vi "Get Property Data (U32).vi"(8 "error in":errorcluster, 10 "Property Name":string, 11 "Item Ref in":refnum<data-value>) -> (0 "error out":errorcluster, 3 "Property Value":u32)   [LabVIEW 2024, in "Config File Parser.lvlib" / "Property.lvclass"]
uses:
  Property.lvclass
  Property.lvclass/Property.ctl
  Item/Item.lvclass
  Property Type.ctl
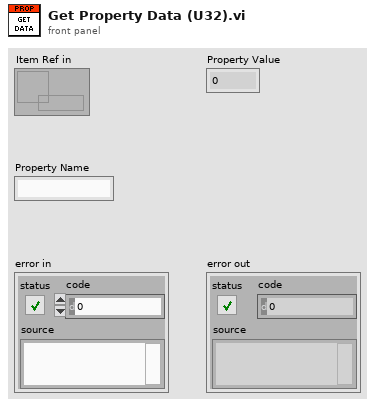
[diagram p1: front panel]
types:
  T1 = typedef "Config File Parser.lvlib/Property.lvclass/Property Type.ctl" = enum16{"Boolean", "Double", "String", "Path", "Dictionary", "DependentFile", "I16", "I32", "I64", "U16", "U32", "U64", "BooleanArray", "DoubleArray", "StringArray", "I16Array", "I32Array", "I64Array", "U16Array", "U32Array", "U64Array"}
  T2 = typedef "Config File Parser.lvlib/Item.lvclass/Item Type.ctl" = enum16{"Property", "Channel", "Section"}
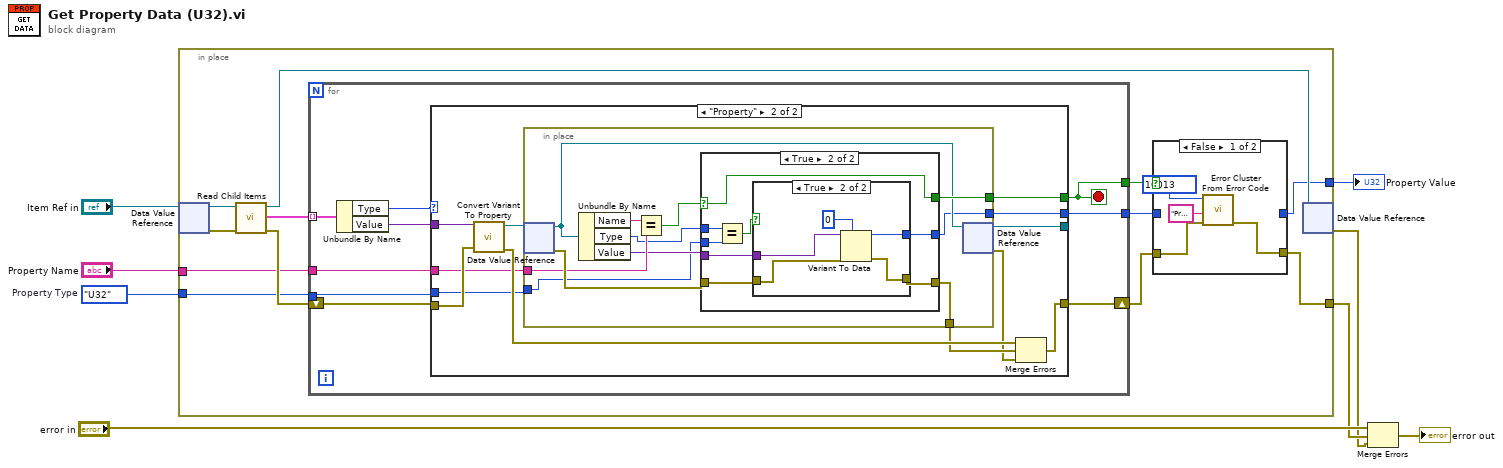
[diagram p0: block diagram]
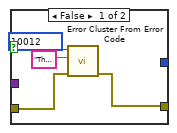
[diagram p5: hidden frame]
diagram:
  w2 = Property_Type."U32"  # Property Type
  n1 = in-place {
    in-place-border: "Property Name" -> [w14]
    in-place-border: w2 -> [w13]
    in-place-border: [w17] -> w7
    in-place-border: [w9] -> w1
    n2 = in-place-dvr #1("Item Ref in") -> (w16:refnum<class "Item.lvclass">, w20:errorcluster)
    n3 = call-dynamic "Read Child Items.vi"("error in"=w20, "Item in"=w16) -> ("error out"=w19:errorcluster, "Child Items"=w15:cluster{"Type":T2, "Value":variant}[], "Item out"=w12:refnum<class "Item.lvclass">)  [unwired: 7 in]
    n4 = for {
      tunnel: w15 -> [w33] mode=indexing
      tunnel: w14 -> [w30]
      tunnel: w13 -> [w29]
      shift-right: [w34] -> w18
      shift-left: w19 -> [w35]
      tunnel: [w28] -> w11
      tunnel: [w27] -> w10
      stop <- w28 stop-if-true
      n5 = Unbundle By Name(w33) -> ("Type"=w32:T2, "Value"=w31:variant)
      n6 = case shown="\"Property\"" w32 {
        tunnel: w31 -> [_ w43]
        tunnel: w30 -> [_ w41]
        tunnel: w29 -> [_ w40]
        tunnel: [_ w39] -> w28
        tunnel: [_ w38] -> _
        tunnel: w35 -> [w36 w48]
        tunnel: [w36 w44] -> w34
        tunnel: [_ w37] -> w27
        frame Default {
        }
        frame "Property" {
          n7 = call "Convert Variant To Property.vi"("error in"=w48, "Property Variant"=w43) -> ("error out"=w47:errorcluster, "Property Ref out"=w42:refnum<data-value>)  [unwired: 8 in]
          n8 = in-place {
            in-place-border: w41 -> [w55]
            in-place-border: w40 -> [w50]
            in-place-border: [w52] -> w39
            in-place-border: [w58] -> w46
            in-place-border: [w49] -> w37
            n9 = in-place-dvr #2(w42) -> (w51:refnum<class "Property.lvclass">, w59:errorcluster)
            n10 = Unbundle By Name(w51) -> ("Name"=w56:string, "Type"=w53:T1, "Value"=w54:variant)
            n11 = Equal?(x=w56, y=w55) -> (x = y?=w57:bool)
            n12 = case shown="True" w57 {
              selector: w57 -> [w60 w62]
              tunnel: [_ w67] -> w49
              tunnel: w54 -> [_ w66]
              tunnel: w50 -> [_ w64]
              tunnel: w53 -> [_ w65]
              tunnel: [w60 w62] -> w52
              tunnel: w59 -> [w61 w69]
              tunnel: [w61 w68] -> w58
              frame False {
              }
              frame True {
                n13 = Equal?(x=w65, y=w64) -> (x = y?=w63:bool)
                n14 = case shown="True" w63 {
                  tunnel: [_ w76] -> w67
                  tunnel: w66 -> [_ w74]
                  tunnel: w69 -> [w73 w78]
                  tunnel: [w72 w77] -> w68
                  frame False {
                    n15 = call <vilib>:"Error Cluster From Error Code.vi"("error in (no error)"=w73, "error message (\"\")"="The selected type is incompatible with the chosen property", "error code (0)"=10012) -> ("error out"=w72:errorcluster)  [unwired: 6 in]
                  }
                  frame True {
                    n16 = Variant To Data(error in=w78, type=u32 0, Variant=w74) -> (data=w76:u32, error out=w77:errorcluster)
                  }
                }
              }
            }
            n17 = in-place-dvr #2(w51) -> (w38:refnum<data-value>, w45:errorcluster)
          }
          n18 = Merge Errors(w47, w46, w45) -> (w44:errorcluster)
        }
      }
    }
    n19 = case shown="False" w11 {
      tunnel: w10 -> [_ w25]
      tunnel: [_ w25] -> w9
      tunnel: w18 -> [w24 w26]
      tunnel: [w23 w26] -> w17
      frame False {
        n20 = call <vilib>:"Error Cluster From Error Code.vi"("error in (no error)"=w24, "error message (\"\")"="Property does not exist", "error code (0)"=10013) -> ("error out"=w23:errorcluster)  [unwired: 6 in]
      }
      frame True {
      }
    }
    n21 = in-place-dvr #1(w12) -> (w6:errorcluster)  [unwired: 1 out]
  }
  "Property Value" <- w1
  n22 = Merge Errors("error in", w7, w6) -> (→"error out":errorcluster)
